vi "Rotate.vi"(8 "error in (no error)":errorcluster, 11 "Log in":refnum<class "Log.lvclass">) -> (0 "error out":errorcluster, 3 "Log out":refnum<class "Log.lvclass">)   [LabVIEW 2026, in "TALOS.lvlib" / "Classes.lvlib" / "Log.lvclass"]
uses:
  Log.lvclass
  Log.lvclass/Log.ctl
  Ancestor/Ancestor/Ancestor.lvclass/Ancestor.ctl
  FGV/Error Memory/Get Error Description.vi
  Support VIs/Get PC name.vi
  Ancestor/Ancestor/Read ID.vi
  Support VIs/Get Class Name.vi
  <vilib>/Utility/error.llb/Clear Errors.vi
  FGV/Error Memory/Error Memory Core.vi
  <vilib>/AdvancedString/Delimited String to 1D String Array.vi
  <vilib>/AdvancedString/Delimited String to 1D String Array (string).vi
  Support VIs/Circus Root Path.vi
  FGV/Error Memory/Error Crt Lvl checker.vi
  FGV/Error Memory/Error Memory Core.vi/40c8088d-b597-4017-91af-faa98e00292e.vi
  FGV/Error Memory/Error Memory Core.vi/d4a3ab98-063c-4e44-b43d-fbdcfe6c2be2.vi
  Support VIs/Global Memory.vi
  <vilib>/Utility/LVClass/Get LV Class Name.vi
  Support VIs/Is in Packed Library.vi
  Support VIs/TALOS Root path.vi
  Support VIs/Read CSV worksheet.vi
  Support VIs/Global Constants.vi
  <vilib>/Utility/error.llb/General Error Handler.vi
  <vilib>/Utility/config.llb/Open Config Data.vi
  <vilib>/Utility/config.llb/Get Section Names.vi
  <vilib>/Utility/config.llb/Get Key Names.vi
  <vilib>/Utility/config.llb/Read Key.vi
  <vilib>/Utility/config.llb/Read Key (String).vi
  <vilib>/Utility/config.llb/Close Config Data.vi
  Ancestor/Ancestor/Ancestor.lvclass
  <vilib>/Comparison/Equal/Equal Functor/Equal Functor.lvclass
  TALOS.lvlib
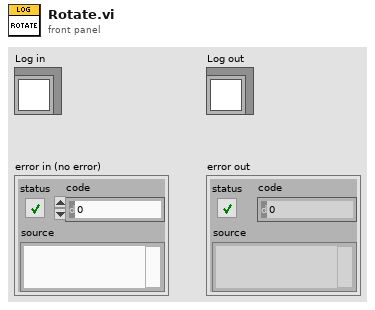
[diagram p1: front panel]
types:
  T1 = enum16{"open", "replace", "create", "open or create", "replace or create", "replace or create with confirmation"}
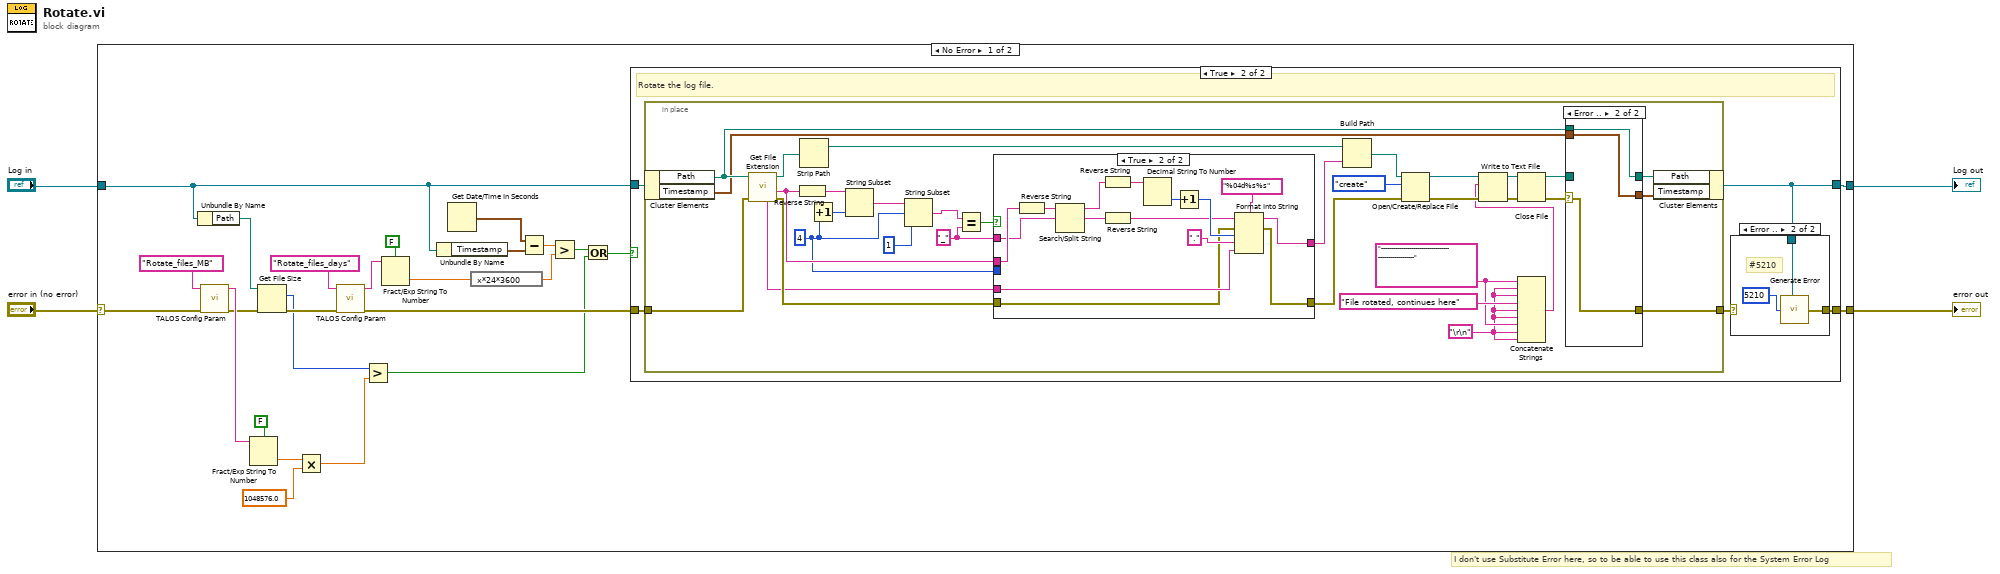
[diagram p0: block diagram]
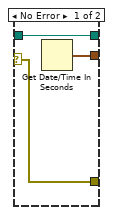
[diagram p4: hidden frame]
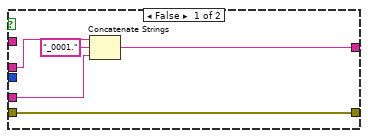
[diagram p5: hidden frame]
diagram:
  # "I don't use Substitute Error here, so to be able to use this class also for the System Error Log"
  n1 = case shown="No Error" "error in (no error)" {
    selector: "error in (no error)" -> [w17 w101]
    tunnel: [w30 w101] -> w4
    tunnel: [w29 w102] -> w2
    tunnel: "Log in" -> [w14 w102]
    frame No Error {
      n2 = Unbundle By Name(w14) -> ("Path"=w13:path)
      n3 = call "TALOS Config Param.vi"("error in (no error)"=w17, "Parameter Name"="Rotate_files_MB") -> ("error out"=w10:errorcluster, "Output"=w15:string)  [unwired: 8 in]
      n4 = Fract/Exp String To Number(use system decimal point (T)=FALSE, string=w15) -> (number=w12:dbl)  [unwired: 2 in, 1 out]
      n5 = Get File Size(file=w13, error in=w10) -> (size (in bytes)=w7:i64, 0:w9:errorcluster)  [unwired: 1 out]
      n6 = Multiply(x=w12, y=1048576.0) -> (x*y=w6:dbl)
      n7 = call "TALOS Config Param.vi"("error in (no error)"=w9, "Parameter Name"="Rotate_files_days") -> ("error out"=w23:errorcluster, "Output"=w21:string)  [unwired: 8 in]
      n8 = Greater?(x=w7, y=w6) -> (0:w5:bool)
      n9 = Fract/Exp String To Number(use system decimal point (T)=FALSE, string=w21) -> (number=w19:dbl)  [unwired: 2 in, 1 out]
      n10 = Unbundle By Name(w14) -> ("Timestamp"=w27:timestamp)
      n11 = Get Date/Time In Seconds() -> (seconds since 1Jan1904=w28:timestamp)
      n12 = expression code="x*24*3600"(w19) -> (w25:dbl)
      n13 = Subtract(x=w28, y=w27) -> (x-y=w26:dbl)
      n14 = Greater?(x=w26, y=w25) -> (0:w24:bool)
      n15 = Or(x=w24, y=w5) -> (x .or. y?=w8:bool)
      n16 = case shown="True" w8 {
        tunnel: [w31 w35] -> w30
        tunnel: w23 -> [w31 w37]
        tunnel: [w32 w34] -> w29
        tunnel: w14 -> [w32 w36]
        frame False {
          # "File recent enough, do nothing."
        }
        frame True {
          # "Rotate the log file."
          n17 = in-place {
            in-place-border: w37 -> [w60]
            in-place-border: [w45] -> w33
            w53 = "----------------------------------------------------"
            w52 = "\r\n"
            w62 = "_" ("y")
            w63 = 4 ("length (rest)")
            n18 = in-place-cluster #1(w36) -> ("Path"=w43:path, "Timestamp"=w42:timestamp)
            n19 = call <vilib>:"Get File Extension.vi"("error in (no error)"=w60, "file"=w43) -> ("error out"=w71:errorcluster, "filename without extension"=w68:string, "dup file"=w72:path, "unmodified file extension"=w69:string)  [unwired: 5 in, 1 out]
            n20 = Reverse String(1:w68) -> (0:w64:string)
            n21 = Strip Path(path=w72) -> (stripped path=w73:path)  [unwired: 1 out]
            n22 = Increment(x=w63) -> (x+1=w70:i32)
            n23 = String Subset(string=w64, length (rest)=w70) -> (substring=w65:string)  [unwired: 1 in]
            n24 = String Subset(string=w65, offset (0)=w63, length (rest)=1 ("length (rest)")) -> (substring=w66:string)
            n25 = Equal?(x=w66, y=w62) -> (x = y?=w67:bool)
            n26 = case shown="True" w67 {
              tunnel: w68 -> [w85 w99]
              tunnel: w69 -> [w83 w90]
              tunnel: [w82 w89] -> w74
              tunnel: w62 -> [_ w98]
              tunnel: w63 -> [_ _]
              tunnel: w71 -> [w81 w88]
              tunnel: [w81 w87] -> w49
              frame False {
                n27 = Concatenate Strings(w85, "_0001." ("string"), w83) -> (w82:string)
              }
              frame True {
                n28 = Reverse String(1:w99) -> (0:w100:string)
                n29 = Search/Split String(string=w100, search string/char (-)=w98) -> (substring before match=w97:string, match + rest of string=w96:string)  [unwired: 1 in, 1 out]
                n30 = Reverse String(1:w97) -> (0:w95:string)
                n31 = Reverse String(1:w96) -> (0:w92:string)
                n32 = Decimal String To Number(string=w95) -> (number=w94:i32)  [unwired: 2 in, 1 out]
                n33 = Increment(x=w94) -> (x+1=w93:i32)
                n34 = Format Into String(format string="%04d%s%s", initial string=w92, error in=w88, w93, "." ("string"), w90) -> (resulting string=w89:string, error out=w87:errorcluster)
              }
            }
            n35 = Build Path(base path=w73, name or relative path=w74) -> (appended path=w50:path)
            n36 = Open/Create/Replace File(file path (use dialog)=w50, error in=w49, operation (0:open)=T1."create") -> (refnum out=w58:refnum<file>, error out=w57:errorcluster)  [unwired: 3 in, 1 out]
            n37 = Concatenate Strings(w53, w52, w52, "File rotated, continues here", w52, w52, w53, w52, w52) -> (w51:string)
            n38 = Write to Text File(file (use dialog)=w58, text=w51, error in=w57) -> (refnum out=w55:refnum<file>, error out=w56:errorcluster)  [unwired: 1 in, 1 out]
            n39 = Close File(refnum=w55, error in=w56) -> (path=w48:path, error out=w47:errorcluster)
            n40 = case shown="Error .." w47 {
              selector: w47 -> [w76 w78]
              tunnel: w48 -> [w77 _]
              tunnel: [w77 w80] -> w46
              tunnel: [w76 w78] -> w45
              tunnel: [w75 w79] -> w44
              tunnel: w43 -> [_ w80]
              tunnel: w42 -> [_ w79]
              frame No Error {
                n41 = Get Date/Time In Seconds() -> (seconds since 1Jan1904=w75:timestamp)
              }
              frame Error {
              }
            }
            n42 = in-place-cluster #1("Path"=w46, "Timestamp"=w44) -> (w34:refnum<class "Log.lvclass">)
          }
          n43 = case shown="Error .." w33 {
            selector: w33 -> [w38 _]
            tunnel: [w38 w40] -> w35
            tunnel: w34 -> [_ w39]
            frame No Error {
            }
            frame Error {
              # "#5210"
              n44 = call "Generate Error.vi"("Class"=w39, "Error Code"=5210) -> ("error out"=w40:errorcluster)  [unwired: 5 in]
            }
          }
        }
      }
    }
    frame Error {
    }
  }
  "error out" <- w4
  "Log out" <- w2
